vi "4339 Create Ch.vi"(8 "sampleRate":dbl=1000.0 format="%0.2f", 10 "Device port info":T1[](array[typedef]), 11 "taskNamesIn":string[](array[string])) -> (0 "error out":errorcluster)   [LabVIEW 2022 SP3]
uses:
  Device ID port info.ctl
  f383c325-543f-44f0-b992-ec9ac167a994.vi
  <vilib>/DAQmx/create/channels.llb/DAQmx Create Channel (AI-Voltage-Custom with Excitation).vi
  <vilib>/DAQmx/create/channels.llb/DAQmx Create Channel (AI-Voltage-Basic).vi
  <vilib>/DAQmx/configure/timing.llb/DAQmx Timing (Sample Clock).vi
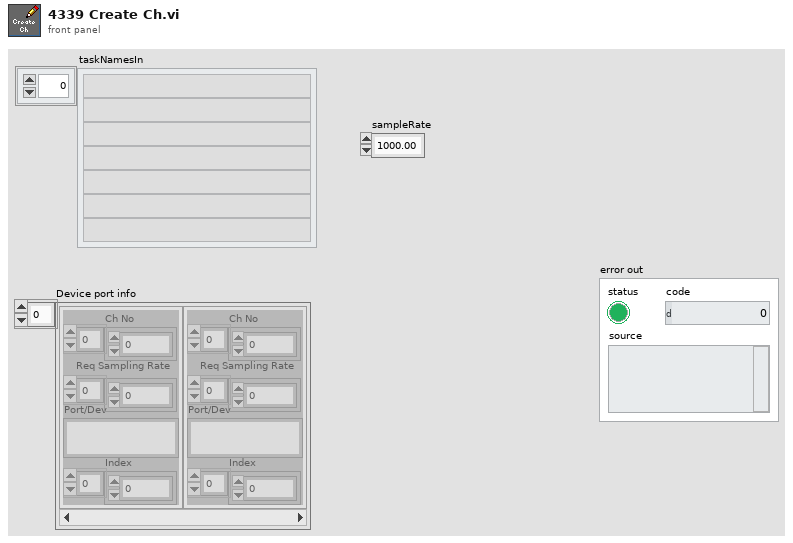
[diagram p1: front panel]
types:
  T1 = typedef "Device ID port info.ctl" = cluster{"Ch No":i16[], "Req Sampling Rate":dbl[], "Port":string, "Index":i32[]}
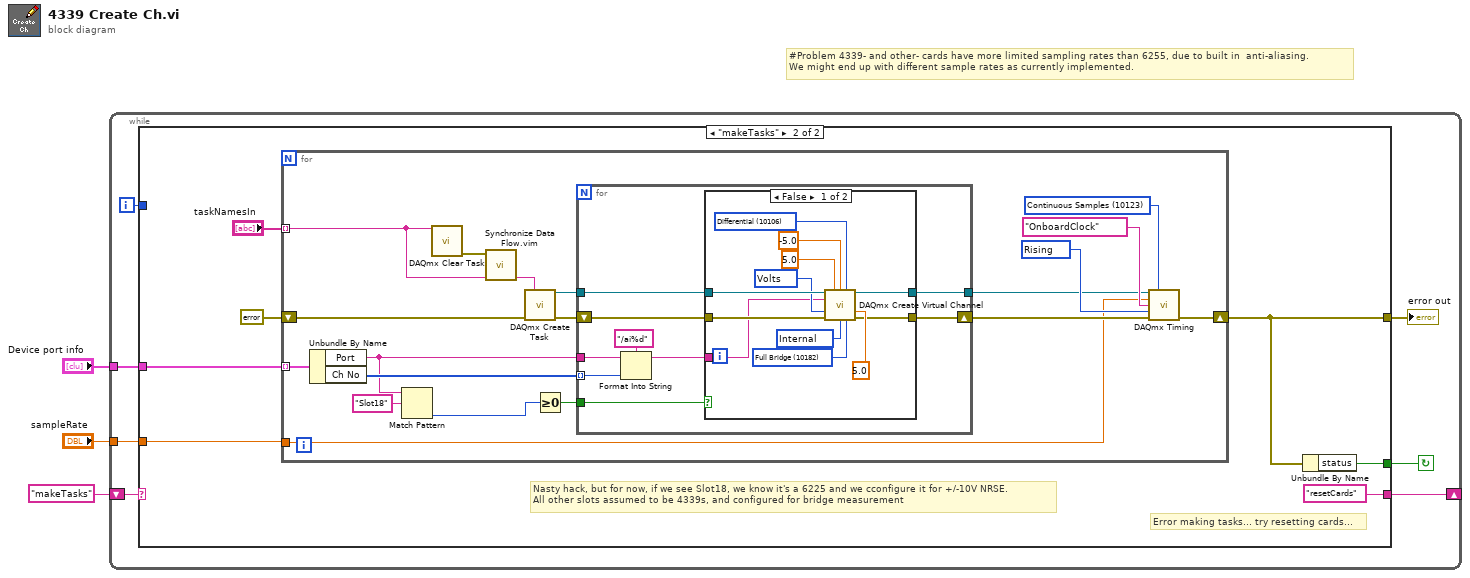
[diagram p0: block diagram]
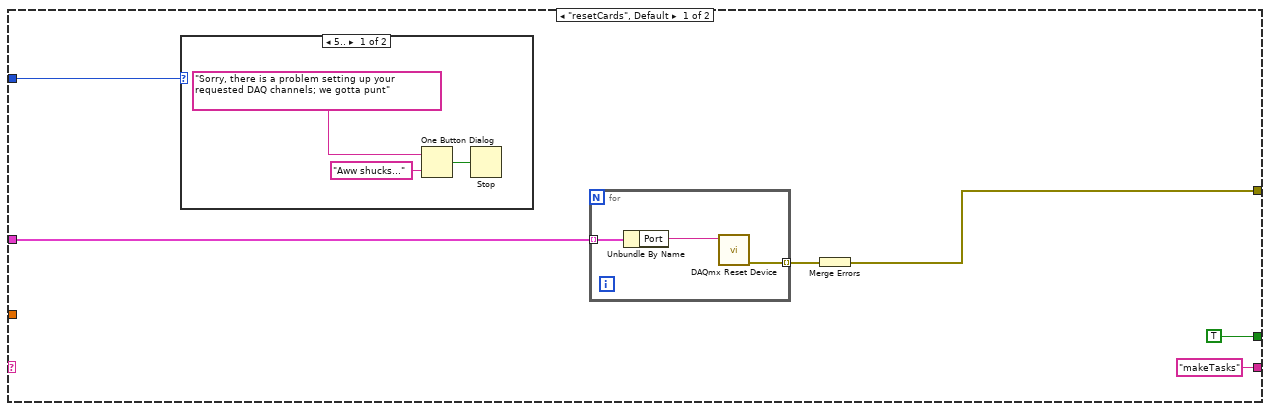
[diagram p2: hidden frame]
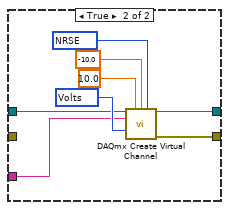
[diagram p4: hidden frame]
diagram:
  # "#Problem 4339- and other- cards have more limited sampling rates than 6255, due to built in  anti-aliasing.\nWe might end up with different sample rates as currently implemented."
  n1 = while {
    tunnel: "Device port info" -> [w10]
    shift-right: [w7] -> _
    shift-left: "makeTasks" -> [w8]
    tunnel: "sampleRate" -> [w6]
    i -> [w5]
    stop <- w9 continue-if-true
    n2 = case shown="\"makeTasks\"" w8 {
      tunnel: w10 -> [w13 w29]
      tunnel: [TRUE w25] -> w9
      tunnel: ["makeTasks" "resetCards"] -> w7
      tunnel: w6 -> [_ w26]
      tunnel: w5 -> [w14 _]
      tunnel: [w11 w24] -> w4
      frame "resetCards", Default {
        n3 = case shown="5.." w14 {
          frame 5.. {
            n4 = One Button Dialog(message="Sorry, there is a problem setting up your requested DAQ channels; we gotta punt", button name ("OK")="Aww shucks...") -> (true=w17:bool)
            n5 = Stop(stop? (T)=w17) -> ()
          }
          frame 0, Default {
          }
        }
        n6 = for {
          tunnel: w13 -> [w22] mode=indexing
          tunnel: [w20] -> w12 mode=indexing
          n7 = Unbundle By Name(w22) -> ("Port"=w21:string)
          n8 = call <vilib>:"DAQmx Reset Device.vi"("device in"=w21) -> ("error out"=w20:errorcluster)  [unwired: 14 in]
        }
        n9 = Merge Errors(w12) -> (w11:errorcluster)
      }
      frame "makeTasks" {
        # "Error making tasks... try resetting cards..."
        # "Nasty hack, but for now, if we see Slot18, we know it's a 6225 and we cconfigure it for +/-10V NRSE.\nAll other slots assumed to be 4339s, and configured for bridge measurement"
        n10 = for {
          tunnel: w29 -> [w47] mode=indexing
          shift-right: [w39] -> w24
          shift-left: errorcluster {"status"=FALSE, "code"=0, "source"=""} ("error out") -> [w48]
          tunnel: w26 -> [w37]
          tunnel: "taskNamesIn" -> [w30] mode=indexing
          w42 = 10280 items=["Rising"=10280, "Falling"=10171] ("active edge")
          w44 = 10123 items=["Finite Samples"=10178, "Continuous Samples"=10123, "Hardware Timed Single Point"=12522] ("sample mode")
          n11 = Unbundle By Name(w47) -> ("Port"=w36:string, "Ch No"=w38:i16[])
          n12 = Match Pattern(string=w36, regular expression="Slot18") -> (offset past match=w34:i32)  [unwired: 1 in, 3 out]
          n13 = call <vilib>:"DAQmx Clear Task.vi"("task in"=w30) -> ("error out"=w32:errorcluster)  [unwired: 14 in]
          n14 = call "Synchronize Data Flow.vim"("input 4"=w30, "input 1"=w32) -> ("output 4"=w31:string)  [unwired: 2 in, 3 out]
          n15 = call <vilib>:"DAQmx Create Task.vi"("new task name"=w31, "error in"=w48) -> ("task out"=w46:refnum<k21>, "error out"=w45:errorcluster)  [unwired: 3 in, 9 out]
          n16 = Greater Or Equal To 0?(x=w34) -> (x >= 0?=w33:bool)
          n17 = for {
            shift-right: [w52] -> w40
            shift-left: w45 -> [w55]
            tunnel: w36 -> [w51]
            tunnel: w38 -> [w50] mode=indexing
            tunnel: w33 -> [w49]
            tunnel: w46 -> [w56]
            tunnel: [w53] -> w41
            n18 = Format Into String(format string="/ai%d", initial string=w51, w50) -> (resulting string=w54:string)  [unwired: 1 in, 1 out]
            n19 = case shown="False" w49 {
              tunnel: w56 -> [w69 w71]
              tunnel: w55 -> [w64 _]
              tunnel: w54 -> [w60 w70]
              tunnel: [w59 w73] -> w53
              tunnel: [w58 w72] -> w52
              frame False {
                w62 = 10182 items=["Full Bridge"=10182, "Half Bridge"=10187, "Quarter Bridge"=10270, "No Bridge"=10228] ("bridge configuration")
                w63 = 10200 items=["Internal"=10200, "External"=10167, "None"=10230] ("voltage excitation source")
                w65 = 10348 items=["Volts"=10348, "From Custom Scale"=10065] ("units")
                w68 = 10106 items=["Default"=-1, "RSE"=10083, "NRSE"=10078, "Differential"=10106, "Pseudodifferential"=12529] ("input terminal configuration")
                n20 = call-poly <vilib>:"DAQmx Create Virtual Channel.vi"("task in"=w69, "maximum value"=5.0, "minimum value"=-5.0, "input terminal configuration"=w68, "physical channels"=w60, "units"=w65, "voltage excitation value"=5.0, "error in"=w64, "voltage excitation source"=w63, "bridge configuration"=w62) -> ("task out"=w59:refnum<k21>, "error out"=w58:errorcluster)  [unwired: 3 in, 1 out]
              }
              frame True {
                w74 = 10348 items=["Volts"=10348, "From Custom Scale"=10065] ("units")
                w77 = 10078 items=["Default"=-1, "RSE"=10083, "NRSE"=10078, "Differential"=10106, "Pseudodifferential"=12529] ("input terminal configuration")
                n21 = call-poly <vilib>:"DAQmx Create Virtual Channel.vi"("task in"=w71, "maximum value"=10.0, "minimum value"=-10.0, "input terminal configuration"=w77, "physical channels"=w70, "units"=w74) -> ("task out"=w73:refnum<k21>, "error out"=w72:errorcluster)  [unwired: 3 in, 5 out]
              }
            }
          }
          n22 = call-poly <vilib>:"DAQmx Timing.vi"("task/channels in"=w41, "sample mode"=w44, "rate"=w37, "source"=tag "OnboardClock", "active edge"=w42, "error in"=w40) -> ("error out"=w39:errorcluster)  [unwired: 1 in, 8 out]
        }
        n23 = Unbundle By Name(w24) -> ("status"=w25:bool)
      }
    }
    "error out" <- w4
  }
